vi "Determine Disabled.vi"(10 "Values in":dbl[](array[numeric]), 11 "Frame Settings in":T1 {"Protection Configurations"."CRC Channels"."Data Type" items=["Signed", "Unsigned", "IEEE Float"]}) -> (1 "Disabled?":bool, 2 "Values out":dbl[](array[numeric]), 3 "Frame Settings out":T1 {"Protection Configurations"."CRC Channels"."Data Type" items=["Signed", "Unsigned", "IEEE Float"]})   [LabVIEW 2023, in "Protection and Counter Support Engine.lvlib"]
uses:
  Protection and Counter Support Engine.lvlib
  Types/RT Frame Settings.ctl
  Shared/Types/Exported Frame Type.ctl
  Types/RT Protection Configuration.ctl
  Shared/Types/Protection Type.ctl
  Shared/Types/XNET Signal Configuration.ctl
  Shared/Types/Exported Counter Settings.ctl
  Shared/Types/Exported Event Trigger Type.ctl
  Shared/Protection and Counter Support Shared.lvlib
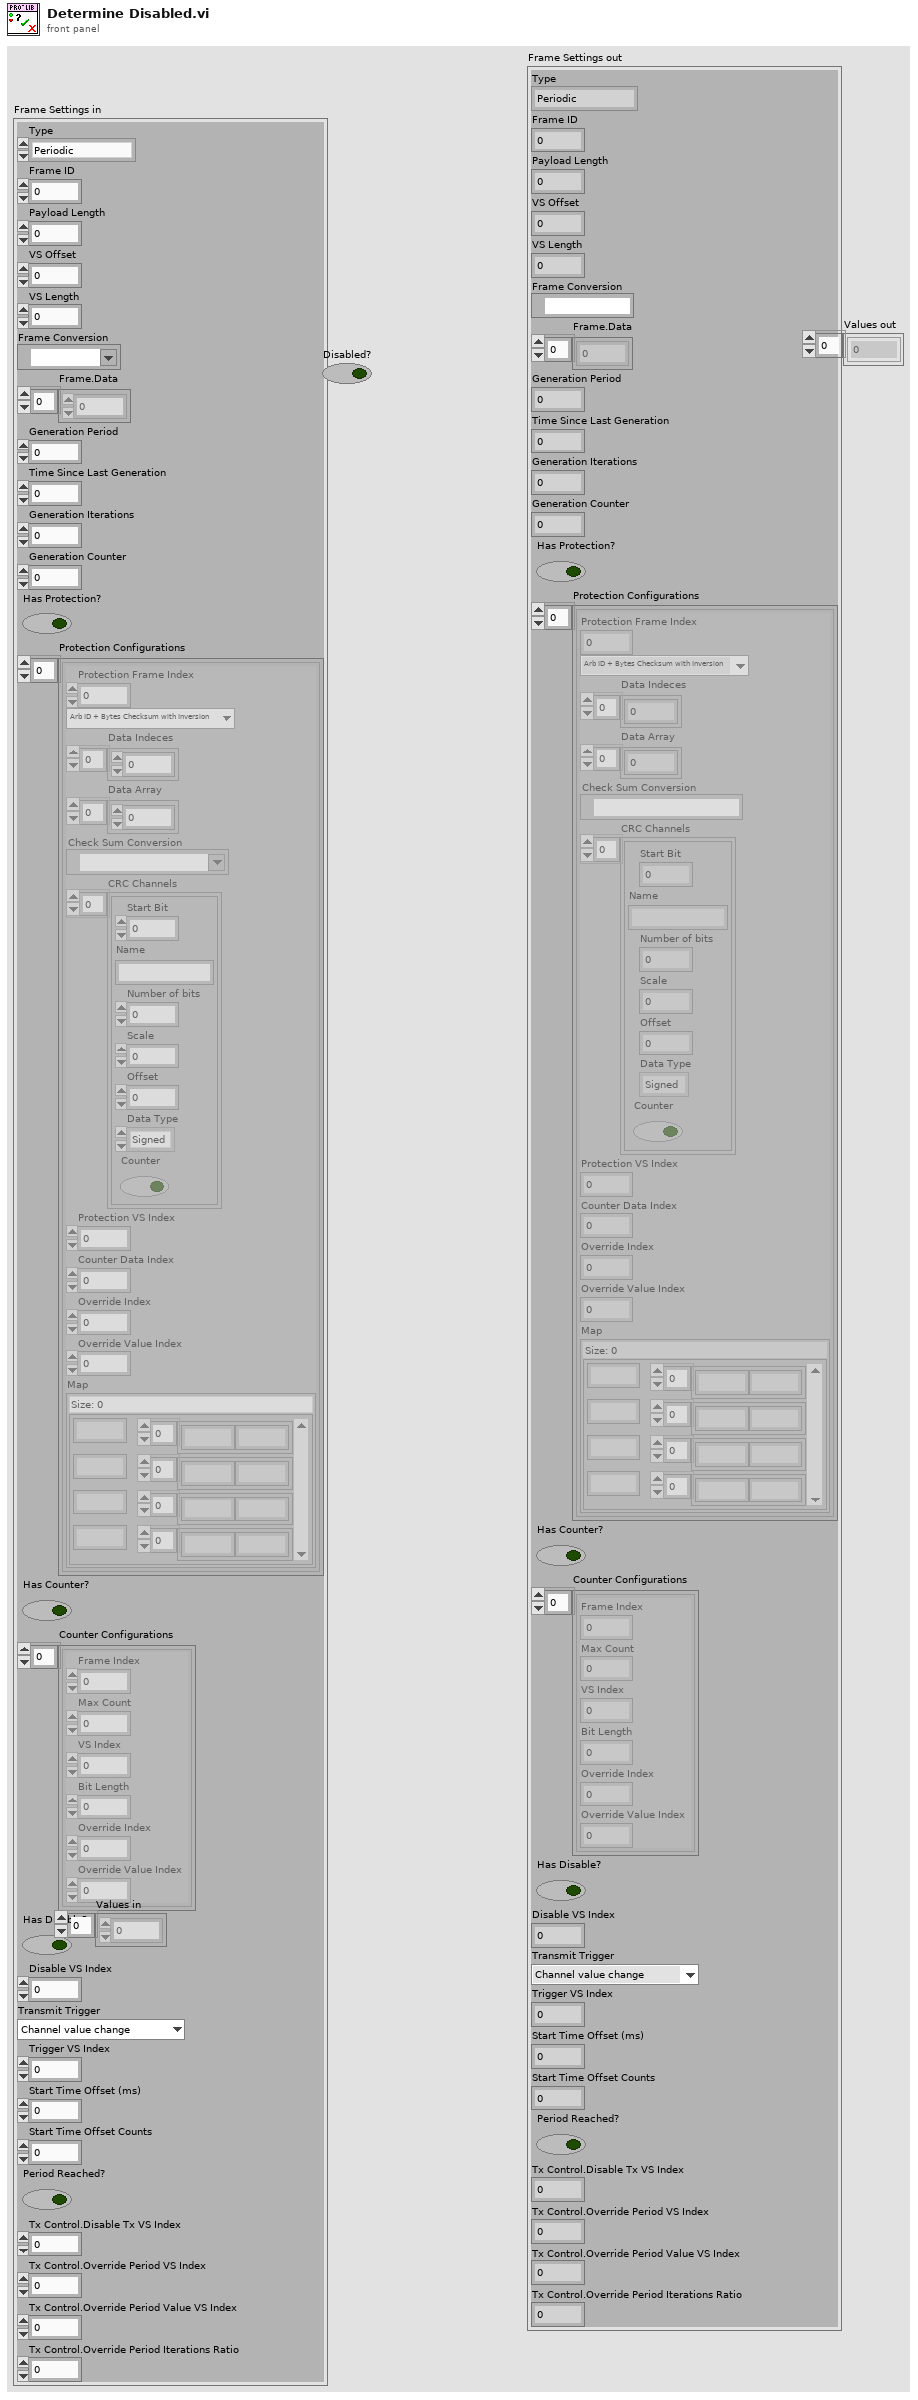
[diagram p1: front panel]
types:
  T1 = typedef "Protection and Counter Support Engine.lvlib/RT Frame Settings.ctl" = cluster{"Type":T2, "Frame ID":u32, "Payload Length":u32, "VS Offset":i32, "VS Length":i32, "Frame Conversion":refnum<k21>, "Frame.Data":dbl[], "Generation Period":u32, "Time Since Last Generation":u32, "Generation Iterations":u32, "Generation Counter":u32, "Has Protection?":bool, "Protection Configurations":T3[], "Has Counter?":bool, "Counter Configurations":T6[], "Has Disable?":bool, "Disable VS Index":i32, "Transmit Trigger":T7, "Trigger VS Index":i32, "Start Time Offset (ms)":u32, "Start Time Offset Counts":u32, "Period Reached?":bool, "Tx Control.Disable Tx VS Index":i32, "Tx Control.Override Period VS Index":i32, "Tx Control.Override Period Value VS Index":i32, "Tx Control.Override Period Iterations Ratio":u32}
  T2 = typedef "Protection and Counter Support Shared.lvlib/Exported Frame Type.ctl" = enum16{"Periodic", "Event", "Periodic/Event"}
  T3 = typedef "Protection and Counter Support Engine.lvlib/RT Protection Configuration.ctl" = cluster{"Protection Frame Index":i32, "Protection Type":T4, "Data Indeces":i32[], "Data Array":dbl[], "Check Sum Conversion":refnum<k21>, "CRC Channels":T5[], "Protection VS Index":i32, "Counter Data Index":i32, "Override Index":i32, "Override Value Index":i32, "Map":map{i32, u8[]}}
  T4 = typedef "Protection and Counter Support Shared.lvlib/Protection Type.ctl" = enum16{"Arb ID + Bytes Checksum with Inversion", "Arb ID + Bytes CRC with Inversion", "Reversed Raw Signal Checksum with Inversion", "Concatenated Two's Compliment", "LP_CRC8", "LP_Checksum", "LP_CRC8_MRS"}
  T5 = typedef "Protection and Counter Support Shared.lvlib/XNET Signal Configuration.ctl" = cluster{"Start Bit":i32, "Name":string, "Number of bits":i32, "Scale":dbl, "Offset":dbl, "Data Type":u32, "Counter":bool}
  T6 = typedef "Protection and Counter Support Shared.lvlib/Exported Counter Settings.ctl" = cluster{"Frame Index":i32, "Max Count":dbl, "VS Index":i32, "Bit Length":i64, "Override Index":i32, "Override Value Index":i32}
  T7 = typedef "Protection and Counter Support Shared.lvlib/Exported Event Trigger Type.ctl" = enum16{"Channel value change", "Trigger channel (not zero)", "Channel value change or trigger channel (not zero)", "Trigger channel (any value change)", "Channel value change or trigger channel (any value change)"}
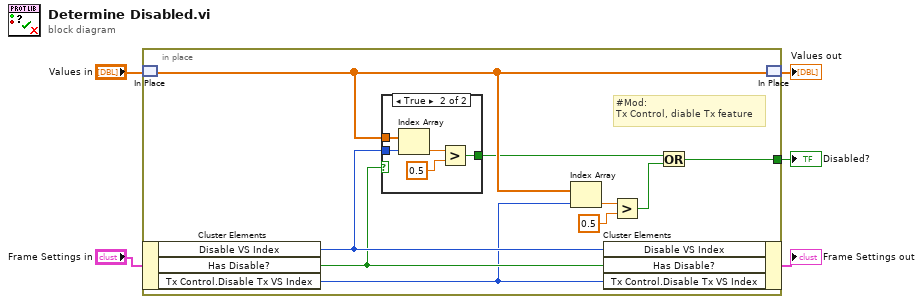
[diagram p0: block diagram]
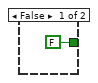
[diagram p2: hidden frame]
diagram:
  n1 = in-place {
    in-place-border: [w6] -> w5
    # "#Mod:\nTx Control, diable Tx feature"
    n2 = in-place-match #1("Values in") -> (w10:dbl[])
    n3 = in-place-cluster #2("Frame Settings in") -> ("Disable VS Index"=w14:i32, "Has Disable?"=w13:bool, "Tx Control.Disable Tx VS Index"=w9:i32)
    n4 = case shown="True" w13 {
      tunnel: w14 -> [_ w20]
      tunnel: w10 -> [_ w19]
      tunnel: [FALSE w17] -> w7
      frame False {
      }
      frame True {
        n5 = Index Array(array=w19, index=w20) -> (element=w18:dbl)
        n6 = Greater?(x=w18, y=0.5 ("x")) -> (0:w17:bool)
      }
    }
    n7 = Index Array(array=w10, index=w9) -> (element=w12:dbl)
    n8 = in-place-cluster #2("Disable VS Index"=w14, "Has Disable?"=w13, "Tx Control.Disable Tx VS Index"=w9) -> (→"Frame Settings out":T1)
    n9 = Greater?(x=w12, y=0.5 ("x")) -> (0:w8:bool)
    n10 = Or(x=w7, y=w8) -> (x .or. y?=w6:bool)
    n11 = in-place-match #1(w10) -> (→"Values out":dbl[])
  }
  "Disabled?" <- w5
